vi "Total数据读取.vi"(0 "configuration file path":path caption="配置文件的路径") -> (7 "Total数值":string)   [LabVIEW 2011]
uses:
  <vilib>/Utility/config.llb/NI_LVConfig.lvlib
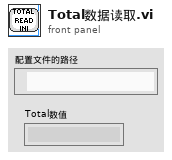
[diagram p1: front panel]
types:
  T1 = typedef "NI_LVConfig.lvlib/Config Data RefNum.ctl" = refnum<k1>
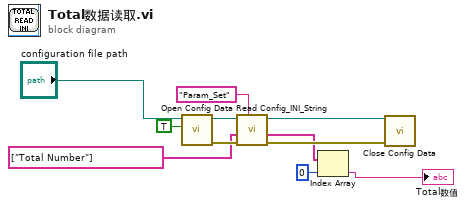
[diagram p0: block diagram]
diagram:
  n1 = call <vilib>:"Open Config Data.vi"("create file if necessary (T)"=TRUE, "configuration file path"="configuration file path") -> ("error out"=w8:errorcluster, "refnum"=w9:T1)  [unwired: 7 in, 1 out]
  n2 = call "Read Config_INI_String.vi"("section"="Param_Set", "error in (no error)"=w8, "Keys"=string[] ["Total Number"], "refnum"=w9) -> ("error out"=w5:errorcluster, "Outputs"=w3:string[], "refnum out"=w6:T1)  [unwired: 5 in]
  n3 = Index Array(array=w3, index=0 ("索引")) -> (element=→"Total数值":string)
  n4 = call <vilib>:"Close Config Data.vi"("error in (no error)"=w5, "refnum"=w6) -> ()  [unwired: 8 in, 2 out]
